vi "renderVideoPage.vi"(8 "error in (no error)":errorcluster, 10 "VideoId":string, 11 "YoutuberDownloader in":refnum<class "YoutuberDownloader.lvclass">) -> (0 "error out":errorcluster, 3 "YoutuberDownloader out":refnum<class "YoutuberDownloader.lvclass">)   [LabVIEW 2018, in "YoutuberDownloader.lvclass"]
uses:
  YoutuberDownloader.lvclass
  ConsoleOut/Print Options.ctl
  YoutuberDownloader.lvclass/YoutuberDownloader.ctl
  Video Class/Video.lvclass/Video.ctl
  ThirdPartyYoutubeLib Class/ThirdPartyYoutubeLib.lvclass
  Video Class/Video.lvclass
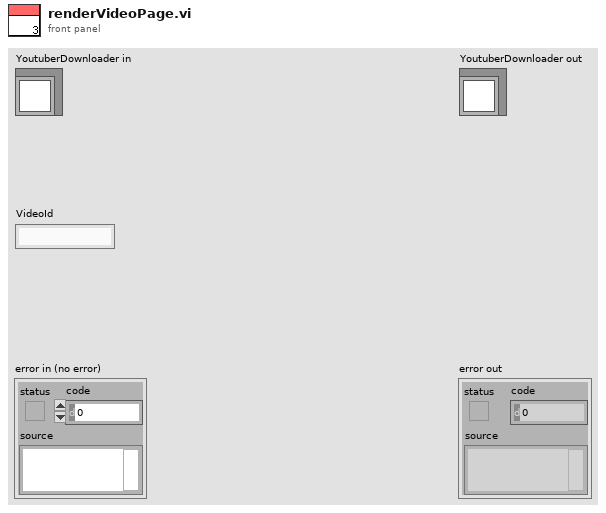
[diagram p1: front panel]
types:
  T1 = typedef "Print Options.ctl" = enum16{"Create", "Get Reference", "Print", "Print Header", "Close"}
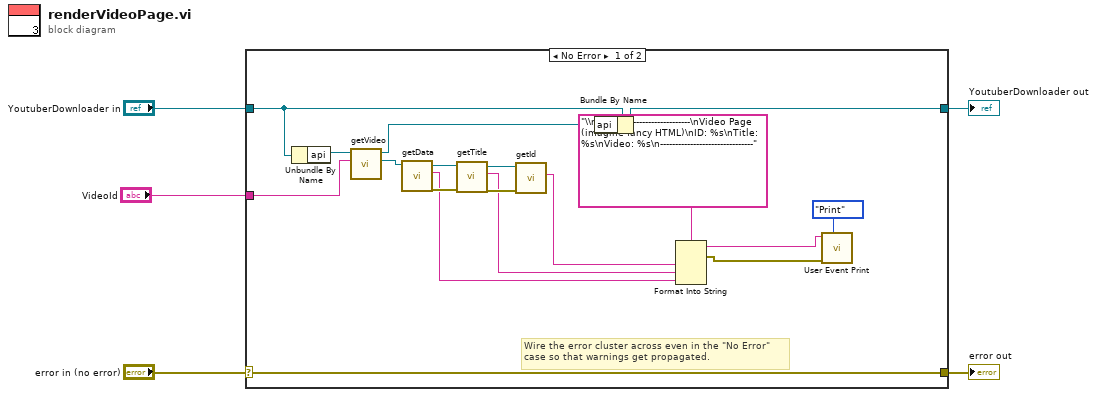
[diagram p0: block diagram]
diagram:
  n1 = case shown="No Error" "error in (no error)" {
    selector: "error in (no error)" -> [w23 w25]
    tunnel: [w23 w25] -> w4
    tunnel: [w7 w24] -> w2
    tunnel: "YoutuberDownloader in" -> [w22 w24]
    tunnel: "VideoId" -> [w20 _]
    frame No Error {
      # "Wire the error cluster across even in the \"No Error\"\ncase so that warnings get propagated."
      n2 = Unbundle By Name(w22) -> ("api"=w21:refnum<class "ThirdPartyYoutubeLib.lvclass">)
      n3 = call-dynamic "getVideo.vi"("Video Id"=w20, "ThirdPartyYoutubeLib in"=w21) -> ("Video"=w14:refnum<class "Video.lvclass">, "ThirdPartyYoutubeLib out"=w6:refnum<class "ThirdPartyYoutubeLib.lvclass">)  [unwired: 7 in, 1 out]
      n4 = call "getData.vi"("Video in"=w14) -> ("error out"=w17:errorcluster, "data"=w13:string, "Video out"=w18:refnum<class "Video.lvclass">)  [unwired: 8 in]
      n5 = call "getTitle.vi"("error in (no error)"=w17, "Video in"=w18) -> ("error out"=w15:errorcluster, "title"=w12:string, "Video out"=w16:refnum<class "Video.lvclass">)  [unwired: 7 in]
      n6 = call "getId.vi"("error in (no error)"=w15, "Video in"=w16) -> ("id"=w11:string)  [unwired: 7 in, 2 out]
      n7 = Bundle By Name(cluster=w22, "api"=w6) -> (w7:refnum<class "YoutuberDownloader.lvclass">)
      n8 = Format Into String(format string="\\n-------------------------------\nVideo Page (imagine fancy HTML)\nID: %s\nTitle: %s\nVideo: %s\n-------------------------------", w11, w12, w13) -> (resulting string=w10:string, error out=w9:errorcluster)  [unwired: 2 in]
      n9 = call "User Event Print.vi"("Options"=Print_Options."Print", "error in (no error)"=w9, "String to Print"=w10) -> ()  [unwired: 7 in, 2 out]
    }
    frame Error {
    }
  }
  "error out" <- w4
  "YoutuberDownloader out" <- w2
